vi "Get LCVR Temperature.vi"(11 "USB Open Device Cluster":T1) -> (3 "Current temp":dbl format="%#_3f")   [LabVIEW 2012]
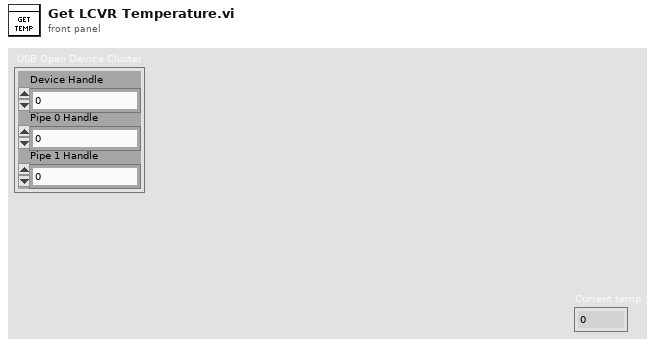
[diagram p1: front panel]
types:
  T1 = cluster{"Device Handle":u32, "Pipe 0 Handle":u32, "Pipe 1 Handle":u32}
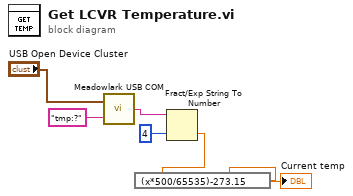
[diagram p0: block diagram]
diagram:
  n1 = call <instrlib>:"Meadowlark USB COM.vi"("WRITE IN String"="tmp:?", "USB Open Device Cluster"="USB Open Device Cluster") -> ("READ OUT String"=w5:string)
  n2 = Fract/Exp String To Number(string=w5, offset=4) -> (number=w3:dbl)  [unwired: 2 in, 1 out]
  n3 = expression code="(x*500/65535)-273.15"(w3) -> (→"Current temp":dbl)
